vi "test json to variant time.vi"(8 "error in (no error)":errorcluster) -> (0 "error out":errorcluster)   [LabVIEW 2019, in "labview_json_tests.lvlib"]
uses:
  labview_json_tests.lvlib
  lib/labview_json.lvlib
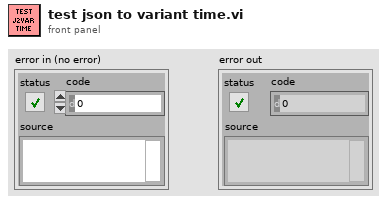
[diagram p1: front panel]
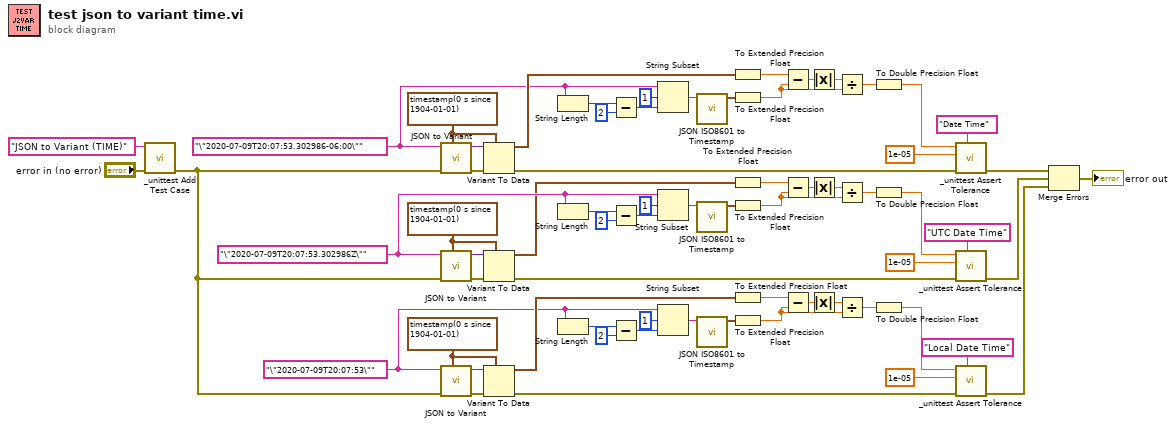
[diagram p0: block diagram]
diagram:
  w4 = timestamp(0 s since 1904-01-01)
  w21 = "\"2020-07-09T20:07:53\""
  w60 = timestamp(0 s since 1904-01-01)
  w61 = timestamp(0 s since 1904-01-01)
  w24 = "\"2020-07-09T20:07:53.302986Z\""
  w42 = "\"2020-07-09T20:07:53.302986-06:00\""
  n1 = call "_unittest Add Test Case.vi"("error in (no error)"="error in (no error)", "Test Case"="JSON to Variant (TIME)") -> ("error out"=w1:errorcluster)  [unwired: 9 in]
  n2 = call "JSON to Variant.vi"("Variant Type"=w61, "error in (no error)"=w1, "JSON"=w42) -> ("error out"=w65:errorcluster, "Variant out"=w62:variant)  [unwired: 7 in]
  n3 = call "JSON to Variant.vi"("Variant Type"=w60, "error in (no error)"=w1, "JSON"=w24) -> ("error out"=w64:errorcluster, "Variant out"=w59:variant)  [unwired: 7 in]
  n4 = call "JSON to Variant.vi"("Variant Type"=w4, "error in (no error)"=w1, "JSON"=w21) -> ("error out"=w3:errorcluster, "Variant out"=w5:variant)  [unwired: 7 in]
  n5 = Variant To Data(error in=w65, type=w61, Variant=w62) -> (data=w43:timestamp, error out=w44:errorcluster)
  n6 = Variant To Data(error in=w64, type=w60, Variant=w59) -> (data=w23:timestamp, error out=w26:errorcluster)
  n7 = Variant To Data(error in=w3, type=w4, Variant=w5) -> (data=w22:timestamp, error out=w20:errorcluster)
  n8 = String Length(string=w42) -> (length=w56:i32)
  n9 = String Length(string=w24) -> (length=w29:i32)
  n10 = String Length(string=w21) -> (length=w17:i32)
  n11 = Subtract(x=w56, y=2) -> (x-y=w54:i32)
  n12 = Subtract(x=w29, y=2) -> (x-y=w31:i32)
  n13 = Subtract(x=w17, y=2) -> (x-y=w15:i32)
  n14 = String Subset(string=w42, offset (0)=1, length (rest)=w54) -> (substring=w58:string)
  n15 = String Subset(string=w24, offset (0)=1, length (rest)=w31) -> (substring=w27:string)
  n16 = String Subset(string=w21, offset (0)=1, length (rest)=w15) -> (substring=w19:string)
  n17 = call "JSON ISO8601 to Timestamp.vi"("ISO 8601 Date Time"=w58) -> ("Local Time Stamp"=w53:timestamp)  [unwired: 10 in]
  n18 = call "JSON ISO8601 to Timestamp.vi"("ISO 8601 Date Time"=w27) -> ("Local Time Stamp"=w32:timestamp)  [unwired: 10 in]
  n19 = call "JSON ISO8601 to Timestamp.vi"("ISO 8601 Date Time"=w19) -> ("Local Time Stamp"=w14:timestamp)  [unwired: 10 in]
  n20 = To Extended Precision Float(1:w43) -> (0:w50:ext)
  n21 = To Extended Precision Float(1:w53) -> (0:w49:ext)
  n22 = To Extended Precision Float(1:w23) -> (0:w35:ext)
  n23 = To Extended Precision Float(1:w32) -> (0:w36:ext)
  n24 = To Extended Precision Float(1:w22) -> (0:w11:ext)
  n25 = To Extended Precision Float(1:w14) -> (0:w10:ext)
  n26 = Subtract(x=w50, y=w49) -> (x-y=w52:ext)
  n27 = Subtract(x=w35, y=w36) -> (x-y=w33:ext)
  n28 = Subtract(x=w11, y=w10) -> (x-y=w13:ext)
  n29 = Absolute Value(x=w52) -> (abs(x)=w51:ext)
  n30 = Absolute Value(x=w33) -> (abs(x)=w34:ext)
  n31 = Absolute Value(x=w13) -> (abs(x)=w12:ext)
  n32 = Divide(x=w51, y=w49) -> (x/y=w48:ext)
  n33 = Divide(x=w34, y=w36) -> (x/y=w37:ext)
  n34 = Divide(x=w12, y=w10) -> (x/y=w9:ext)
  n35 = To Double Precision Float(number=w48) -> (double precision float=w45:dbl)
  n36 = To Double Precision Float(number=w37) -> (double precision float=w40:dbl)
  n37 = To Double Precision Float(number=w9) -> (double precision float=w6:dbl)
  n38 = call "_unittest Assert Tolerance.vi"("Message"="Date Time", "error in (no error)"=w44, "Tollerance (1E-5)"=1e-05, "Actual Value"=w45) -> ("error out"=w41:errorcluster)  [unwired: 7 in]
  n39 = call "_unittest Assert Tolerance.vi"("Message"="UTC Date Time", "error in (no error)"=w26, "Tollerance (1E-5)"=1e-05, "Actual Value"=w40) -> ("error out"=w25:errorcluster)  [unwired: 7 in]
  n40 = call "_unittest Assert Tolerance.vi"("Message"="Local Date Time", "error in (no error)"=w20, "Tollerance (1E-5)"=1e-05, "Actual Value"=w6) -> ("error out"=w2:errorcluster)  [unwired: 7 in]
  n41 = Merge Errors(w41, w25, w2) -> (→"error out":errorcluster)
